vi "Error Bound Wait (ms).vi"(6 "milliseconds to wait (100)":u32=100, 8 "error in":errorcluster) -> (0 "error out":errorcluster)   [LabVIEW 2018]
doc: "Wait the specified number of ms unless there is an error."
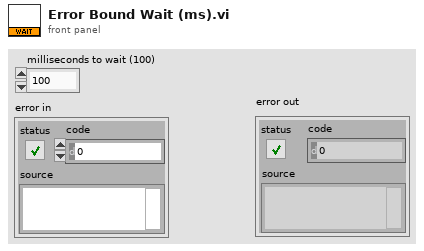
[diagram p1: front panel]
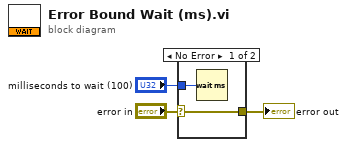
[diagram p0: block diagram]
diagram:
  n1 = case shown="No Error" "error in" {
    selector: "error in" -> [w5 w6]
    tunnel: [w5 w6] -> w2
    tunnel: "milliseconds to wait (100)" -> [w4 _]
    frame No Error {
      n2 = Wait (ms)(milliseconds to wait=w4) -> ()  [unwired: 1 out]
    }
    frame Error {
    }
  }
  "error out" <- w2
